vi "UMLEditor_OptionsDialog.vi"(1 "localVariables":T2 {"ObjectHotspots"."HotSpot"."y" format="%.2f"; "ObjectHotspots"."HotSpot"."x" format="%.2f"; "NodesBounds"."height" format="%.2f"; "NodesBounds"."width" format="%.2f"; "NodesBounds"."y" format="%.2f"; "NodesBounds"."x" format="%.2f"; "offset"."y" format="%.2f"; "offset"."x" format="%.2f"; "gridSize" format="%.2f"; "dragStartBounds"."height" format="%.2f"; "dragStartBounds"."width" format="%.2f"; "dragStartBounds"."y" format="%.2f"; "dragStartBounds"."x" format="%.2f"; "dragStartPoint"."y" format="%.2f"; "dragStartPoint"."x" format="%.2f"; "rubberBandStart"."y" format="%.2f"; "rubberBandStart"."x" format="%.2f"; "lastMousePoint"."y" format="%.2f"; "lastMousePoint"."x" format="%.2f"; "zoom" format="%.2f"}, 5 "error in (no error)":errorcluster) -> (19 "error out":errorcluster)   [LabVIEW 2020]
doc: "Helpinstructions."
uses:
  <resource>/Framework/Providers/Open_GDS/UML/UMLEditor/UMLEditor LocalVariablesType.ctl
  <resource>/Framework/Providers/Open_GDS/UML/AbstractNode_class/AbstractNode.lvclass
  <resource>/Framework/Providers/Open_GDS/UML/Graphics_class/Graphics.lvclass
  <resource>/Framework/Providers/Open_GDS/UML/Grid_class/Grid.lvclass
  <resource>/Framework/Providers/Open_GDS/UML/AbstractEdge_class/AbstractEdge.lvclass
  <resource>/Framework/Providers/Open_GDS/UML/UMLEditor/UMLEditor statesType.ctl
  <resource>/Framework/Providers/Open_GDS/UML/UMLEditor/UMLEditor tooltype.ctl
  <resource>/Framework/Providers/Open_GDS/UML/UMLEditor/UMLEditor_DiagramInfo.ctl
  <resource>/Framework/Providers/Open_GDS/UML/Graph_class/Graph.lvclass
  <resource>/Framework/Providers/Open_GDS/UML/General/Point/Point Point2D.ctl
  <resource>/Framework/Providers/Open_GDS/UML/General/Rectangle/Rectangle Rectangle2D.ctl
  <resource>/Framework/Providers/Open_GDS/UML/UMLEditor/UMLEditor ExportType.ctl
  <resource>/Framework/Providers/Open_GDS/UML/UMLEditor/UMLEditor FlattenCommandType.ctl
  <resource>/Framework/Providers/Open_GDS/UML/UMLEditor/UMLEditor ExecuteCommandType.ctl
  <resource>/Framework/Providers/Open_GDS/UML/ContextHelp/ContextHelp_EventType.ctl
  <resource>/Framework/Providers/Open_GDS/UML/UMLEditor/UMLEditor_HotSpotData.ctl
  <resource>/Framework/Providers/Open_GDS/UML/UMLEditor/UMLEditor_HotSpotType.ctl
  <resource>/Framework/Providers/Open_GDS/UML/UmlEditor_class/EventData.ctl
  <resource>/Framework/Providers/Open_GDS/UML/UMLEditor/UMLEditor_SyncOptions.ctl
  <resource>/Framework/Providers/Open_GDS/ClassProviders/Common/File/File_StoredPathesActions.ctl
  <resource>/Framework/Providers/Open_GDS/UML/UMLEditor/UMLEditor_StoredPathes.ctl
  <resource>/Framework/Providers/Open_GDS/UML/UMLEditor/UMLEditor_StoredColors.ctl
  <resource>/Framework/Providers/Open_GDS/ClassProviders/Common/CommonVIs/CommonVIs_ColorMemoryAction.ctl
  <resource>/Framework/Providers/Open_GDS/UML/ClassNode_class/ClassNode.lvclass
  C:/Program Files (x86)/National Instruments/LabVIEW 2020/resource/Framework/Providers/Open_GDS/UML/AbstractNode_class/AbstractNode.lvclass
  <resource>/Framework/Providers/Open_GDS/UML/ContextHelp/ContextHelp_HelpTexts.ctl
  <resource>/Framework/Providers/Open_GDS/UML/ClassNode_class/ExternalSetTypes.ctl
  <resource>/Framework/Providers/Open_GDS/UML/UmlEditor_class/UmlEditor.lvclass
panel:
  out "TabLabel":string
  out "Tab":enum32{"Color", "Paths", "General", "AutoSync"}(tab)
  in  "Class background color for <<Interface>> Stereotypes":u32(colorbox)
  in  "Default class background":u32(colorbox)
  in  "Class background with path property defined":u32(colorbox)
  in  "Class background color for <<Application/VI>> Stereotypes":u32(colorbox)
  in  "Class background color for <<TYPE/ENUM>> Stereotype":u32(colorbox)
  in  "State Background Color":u32(colorbox)
  in  "UseProjectPath":bool
  in  "ClassBasePath":path caption="Class Base Path\n(Used when releative class pathes is used)"
  in  "Classes":string(tree) caption="These classes could be converted to use a relative path"
  in  "Convert":bool
  in  "VIPath":path caption="Stereotype <<VI>>"
  in  "ApplicationPath":path caption="Stereotype <<Application>> template file"
  in  "NewFilterName":string
  in  "Filter":u16(ring) items=["Custom", "Actore Framework", "-", "Save current filter..."]
  in  "SyncOption":T1
  in  "OpenLastSavedDiagram":bool
  in  "Max number of undo steps":i32=4 min=4 max=20
  in  "ActivateUndo":bool
  in  "Classes to ignore in sychronization":string[][](table)
  in  "Attributes to ignore in sychronization":string[][](table)
  in  "CreateTypes":bool
  in  "_DeleteFilter":bool
  in  "AutoSync":u32=1 caption="Auto Synchronize diagram from source every (s)" min=1 max=3600
  in  "OptionTree":string(tree)
  in  "Help":bool
  out "ClassArray":string[](array[string])
  out "RefArray":refnum<class "AbstractNode.lvclass">[](array[class])
  in  "OK":bool
  in  "Cancel":bool
  # "Class nodes in class diagrams"
  # "State nodes in state diagrams"
  # "Template file"
  # "Note. Empty VIs will be used if template file paths are empty"
  # "Synchronization options for\nclasses and VIs"
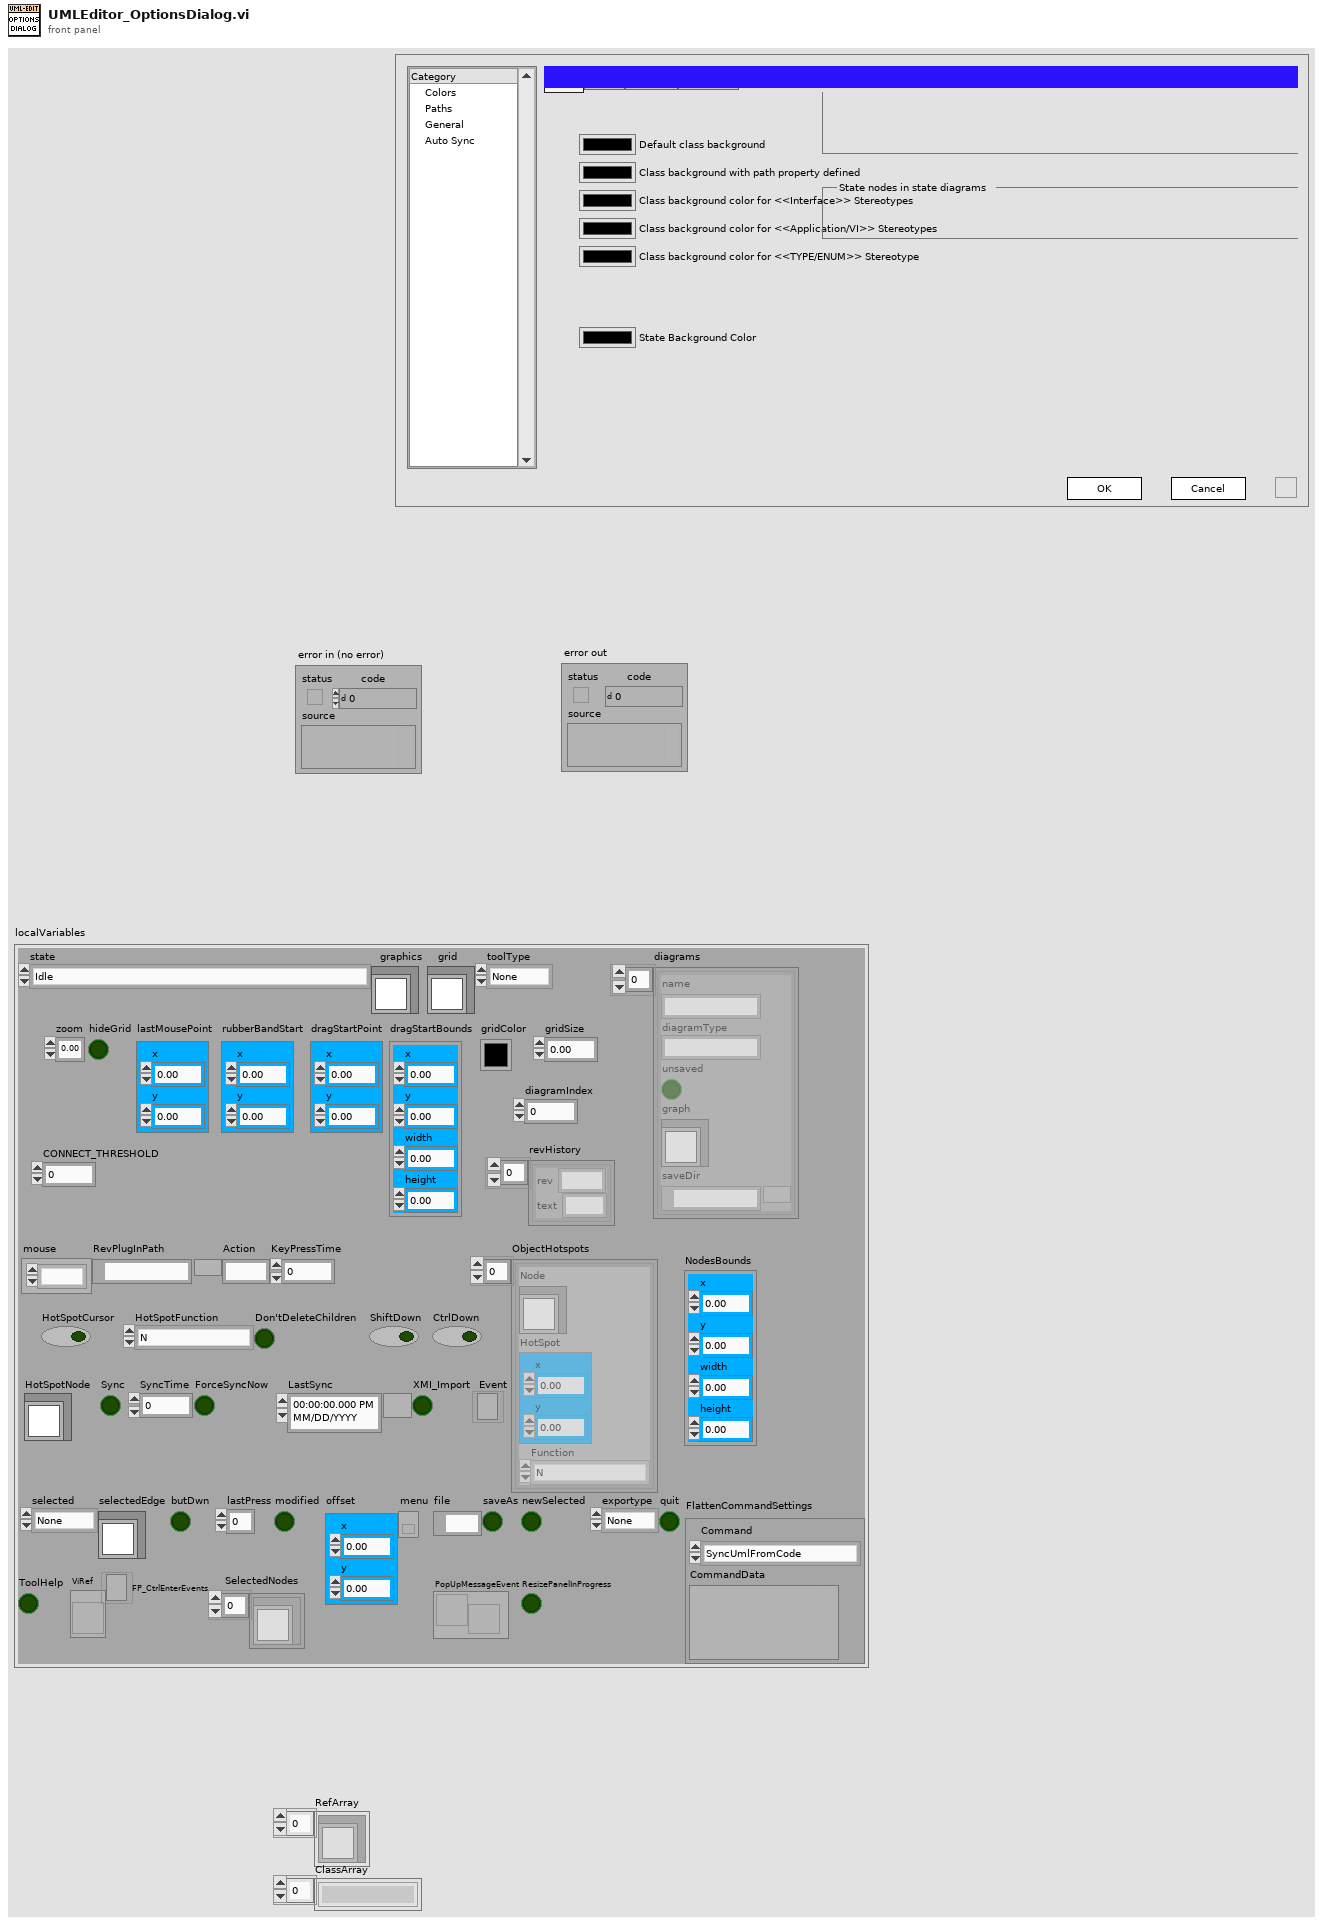
[diagram p1: front panel]
types:
  T1 = typedef "UMLEditor_SyncOptions.ctl" = cluster{"IgnoreInstrLib":bool, "IgnoreUserLib":bool, "IgnoreViLib":bool}
  T2 = typedef "UMLEditor LocalVariablesType.ctl" = cluster{"state":T3, "graphics":refnum<class "Graphics.lvclass">, "grid":refnum<class "Grid.lvclass">, "toolType":T4, "diagramIndex":i32, "diagrams":T5[], "zoom":dbl, "hideGrid":bool, "lastMousePoint":T6, "rubberBandStart":T6, "dragStartPoint":T6, "dragStartBounds":T7, "gridColor":u32, "gridSize":dbl, "CONNECT_THRESHOLD":i32, "selected":T4, "selectedEdge":refnum<class "AbstractEdge.lvclass">, "butDwn":bool, "lastPress":u32, "modified":bool, "offset":T6, "menu":refnum<k9>, "file":path, "saveAs":bool, "newSelected":bool, "exportype":T8, "quit":bool, "revHistory":cluster{"rev":string, "text":string}[], "FlattenCommandSettings":T9, "PopUpMessageEvent":T11, "ResizePanelInProgress":bool, "NodesBounds":T7, "ToolHelp":bool, "ViRef":refnum<vi>, "FP_CtrlEnterEvents":refnum<event-registration>, "SelectedNodes":refnum<class "AbstractNode.lvclass">[], "mouse":refnum<k1>, "RevPlugInPath":path, "Action":string, "KeyPressTime":u32, "ObjectHotspots":T12[], "HotSpotCursor":bool, "HotSpotFunction":T13, "Don'tDeleteChildren":bool, "ShiftDown":bool, "CtrlDown":bool, "HotSpotNode":refnum<class "AbstractNode.lvclass">, "Sync":bool, "SyncTime":u32, "ForceSyncNow":bool, "LastSync":timestamp, "XMI_Import":bool, "Event":refnum<event-registration>}
  T3 = typedef "UMLEditor statesType.ctl" = enum16{"Idle", "CheckLicense", "revHistory", "Init", "Init2", "EditSelected", "RemoveSelected", "PaintComponent", "ChangeZoom", "ChangeGridSize", "Open", "Close", "Save", "ExportPicture", "Export", "Repaint", "Error", "Exit", "QUIT", "CreateScript", "ExecuteScript", "ClassReversedEngineering", "PlugInReverseEngineering", "StateReversedEngineering", "AutoPlace", "ExecuteCommand", "OpenClass", "SyncAll", "StraightenAssociation", "Copy", "Paste", "AddNodeFromProjectTree", "AddNodeFromProjectTree+SyncAll", "PanAndRepaint", "Init3", "CopyPaste", "ApplyDesignPattern", "AnalyseViInStateDiagram", "AutoSync"}
  T4 = typedef "UMLEditor tooltype.ctl" = enum16{"None", "Node", "Edge"}
  T5 = typedef "UMLEditor_DiagramInfo.ctl" = cluster{"name":string, "diagramType":string, "unsaved":bool, "graph":refnum<class "Graph.lvclass">, "saveDir":path}
  T6 = typedef "Point Point2D.ctl" = cluster{"x":dbl, "y":dbl}
  T7 = typedef "Rectangle Rectangle2D.ctl" = cluster{"x":dbl, "y":dbl, "width":dbl, "height":dbl}
  T8 = typedef "UMLEditor ExportType.ctl" = enum16{"None", "Printer", "png", "jpg", "roseUML"}
  T9 = typedef "UMLEditor FlattenCommandType.ctl" = cluster{"Command":T10, "CommandData":variant}
  T10 = typedef "UMLEditor ExecuteCommandType.ctl" = enum16{"SyncUmlFromCode", "SyncCodeFromUML", "OpenClass", "OpenFile", "CreateClass", "CreateVI", "OpenClassAttribute", "LocateInProject", "GraphExecute"}
  T11 = typedef "ContextHelp_EventType.ctl" = refnum<user-event>
  T12 = typedef "UMLEditor_HotSpotData.ctl" = cluster{"Node":refnum<class "AbstractNode.lvclass">, "HotSpot":T6, "Function":T13}
  T13 = typedef "UMLEditor_HotSpotType.ctl" = enum16{"N", "NE", "E", "SE", "S", "SW", "W", "NW", "Expand", "Collaps"}
  T14 = typedef "UMLEditor_StoredColors.ctl" = enum16{"ClassBackgroudColor", "ClassBackgroudColorWithClassPath", "ClassBackgroudColorForApplicationVIStereotype", "ClassBackgroudColorForTypeStereotype", "StateBackgroudColor", "ClassBackgroudColorForInterfaceStereotype"}
  T15 = typedef "UMLEditor_StoredPathes.ctl" = enum16{"LastSearchPath", "QueuedArrayStateVI", "ClassBasePath", "ViTemplatePath", "ApplicationTemplatePath", "IniFilePath", "WizDir", "RevPlugInPath"}
  T16 = typedef "File_StoredPathesActions.ctl" = enum16{"Get Path", "Set Path", "Delete Path", "Clear All Paths"}
  T17 = cluster{"reference out":refnum<class "AbstractNode.lvclass">, "className":string, string, string}[]
  T18 = cluster{"reference out":refnum<class "ClassNode.lvclass">, "className":string, string, string}
  T19 = typedef "ContextHelp_HelpTexts.ctl" = enum16{"None(Hide)", "Default", "Help", "Welcome", "GettingStarted", "ClassDiagram_Help", "SequenceDiagram_Help", "UseCaseDiagram_Help", "BSelect", "BClass", "BInterface", "BPackage", "BNote", "BDependency", "BInheritance", "BInterfaceImplementation", "BAssociation", "BAggregation", "BCompAggregation", "BNoteConnector", "BObject", "BActionBar", "BCall", "BSystem", "BActor", "BUseCase", "BGeneralization", "BIncludes", "BExtends", "BUseCaseDiagramAssociation", "ClassRelationshipEdge editDialog_Bent Style", "ClassRelationshipEdge editDialog_RelationType", "ClassRelationshipEdge editDialog_Reverse association", "ClassRelationshipEdge editDialog_Start label", "ClassRelationshipEdge editDialog_Middle label", "ClassRelationshipEdge editDialog_End label", "UMLEditor reversedEngineering_Pathes", "ReversedEngineering StateReverseDialog_Help", "ReversedEngineering StateQueuedSettings_Help", "UMLEditor reversedEngineering_AddTopVIs", "UMLEditor reversedEngineering_AddClasses", "UMLEditor reversedEngineering_AddDirs", "UMLEditor reversedEngineering_Recursively", "UMLEditor reversedEngineering_Remove", "UMLEditor reversedEngineering_ClearList", "UMLEditor reversedEngineering_HideSubAss", "UMLEditor reversedEngineering_CreateTypes", "UMLEditor reversedEngineering_OnlyInheritance", "UMLEditor reversedEngineering_CreateApplication", "UMLEditor reversedEngineering_OK", "UMLEditor reversedEngineering_Cancel", "UMLEditor reversedEngineering_Help", "UMLEditor createWizardScriptFile_ScriptfilePath", "UMLEditor createWizardScriptFile_ClassPath", "UMLEditor createWizardScriptFile_Use", "UMLEditor createWizardScriptFile_PrivateDirName", "UMLEditor createWizardScriptFile_DirAppend", "UMLEditor createWizardScriptFile_Separator Character", "UMLEditor createWizardScriptFile_OK", "UMLEditor createWizardScriptFile_Cancel", "UMLEditor createWizardScriptFile_Help", "ClassNode editDialog_Class Name", "InterfaceNode editDialog_Class Name", "ClassNode editDialog_Attribute", "ClassNode editDialog_Methods", "InterfaceNode editDialog_Methods", "ClassNode editDialog_connection", "InterfaceNode editDialog_connection", "ClassNode editDialog_StereoType", "ClassNode editDialog_ShowAttrib", "ClassNode editDialog_ShowMethods", "ClassNode editDialog_ClassPath", "ClassNode editDialog_AddAttribute", "ClassNode editDialog_AddMethod", "InterfaceNode editDialog_AddMethod", "ClassNode AttributeGuide_AttributeName", "ClassNode AttributeGuide_Array?", "ClassNode AttributeGuide_Data Type", "ClassNode AttributeGuide_RefName", "ClassNode AttributeGuide_Preview", "ClassNode AttributeGuide_OK", "ClassNode AttributeGuide_Cancel", "ClassNode MethodGuide_Visibility", "ClassNode MethodGuide_Method Name", "ClassNode MethodGuide_Preview", "ClassNode MethodGuide_OK", "ClassNode MethodGuide_Cancel", "CallNode EditCallProperties_AllButtons", "ObjectNode EditObjectlProperties_AllButtons", "ActorNode EditActorProperties_AllButtons", "UseCaseRelationshipNode EditUseCaselProperties_AllButtons", "UseCaseNode EditUseCaselProperties_AllButtons", "SystemNode EditSystemProperties_AllButtons", "ReversedEngineering UpdateAttributes_AllButtons", "StateNode editDialog_AllButtons", "StateTransition editDialog_AllButtons", "ArrangeNodes Main_Picture", "ArrangeNodes Main_Zoom", "ArrangeNodes Main_Auto Zoom", "ArrangeNodes Main_shorten", "ArrangeNodes Main_Min Length", "ArrangeNodes Main_Max Length", "ArrangeNodes Main_increase", "ArrangeNodes Main_decrease", "ArrangeNodes Main_Shake", "ArrangeNodes Main", "BState", "BInitialState", "BFinalState", "BStateTransition", "StateDiagram_Help", "StateDiagram_PropertiesAllButtons", "ReversedEngineering StateReverseDialog_ClearStates", "ReversedEngineering StateReverseDialog_UseQueuedStateMachines", "ReversedEngineering StateReverseDialog_QueuedSettings", "ReversedEngineering StateReverseDialog_SearchForVIs", "ReversedEngineering StateReverseDialog_SearchCriteria", "OptionsDialog_ClassBasePath", "OptionsDialog_VIPath", "OptionsDialog_ApplicationPath", "OptionsDialog_WizDir", "OptionsDialog_IniFilePath", "OptionsDialog_DefineColors", "OptionsDialog_Help", "OptionsDialog_CreateTypes", "ClassRelationshipEdge editDialog_SplitWire"}
  T20 = typedef "ClassNode.lvclass/ExternalSetTypes.ctl" = enum16{"Name", "Attributes", "Methods", "Position", "ShowMethods", "ShowAttributes", "ClassPath"}
  T21 = typedef "CommonVIs_ColorMemoryAction.ctl" = enum16{"Get Color", "Set Color", "Delete Color", "Clear All Colors"}
  T22 = typedef "ContextHelp_ShowType.ctl" = cluster{"Header":string, "Picture":picture, "Text":string}
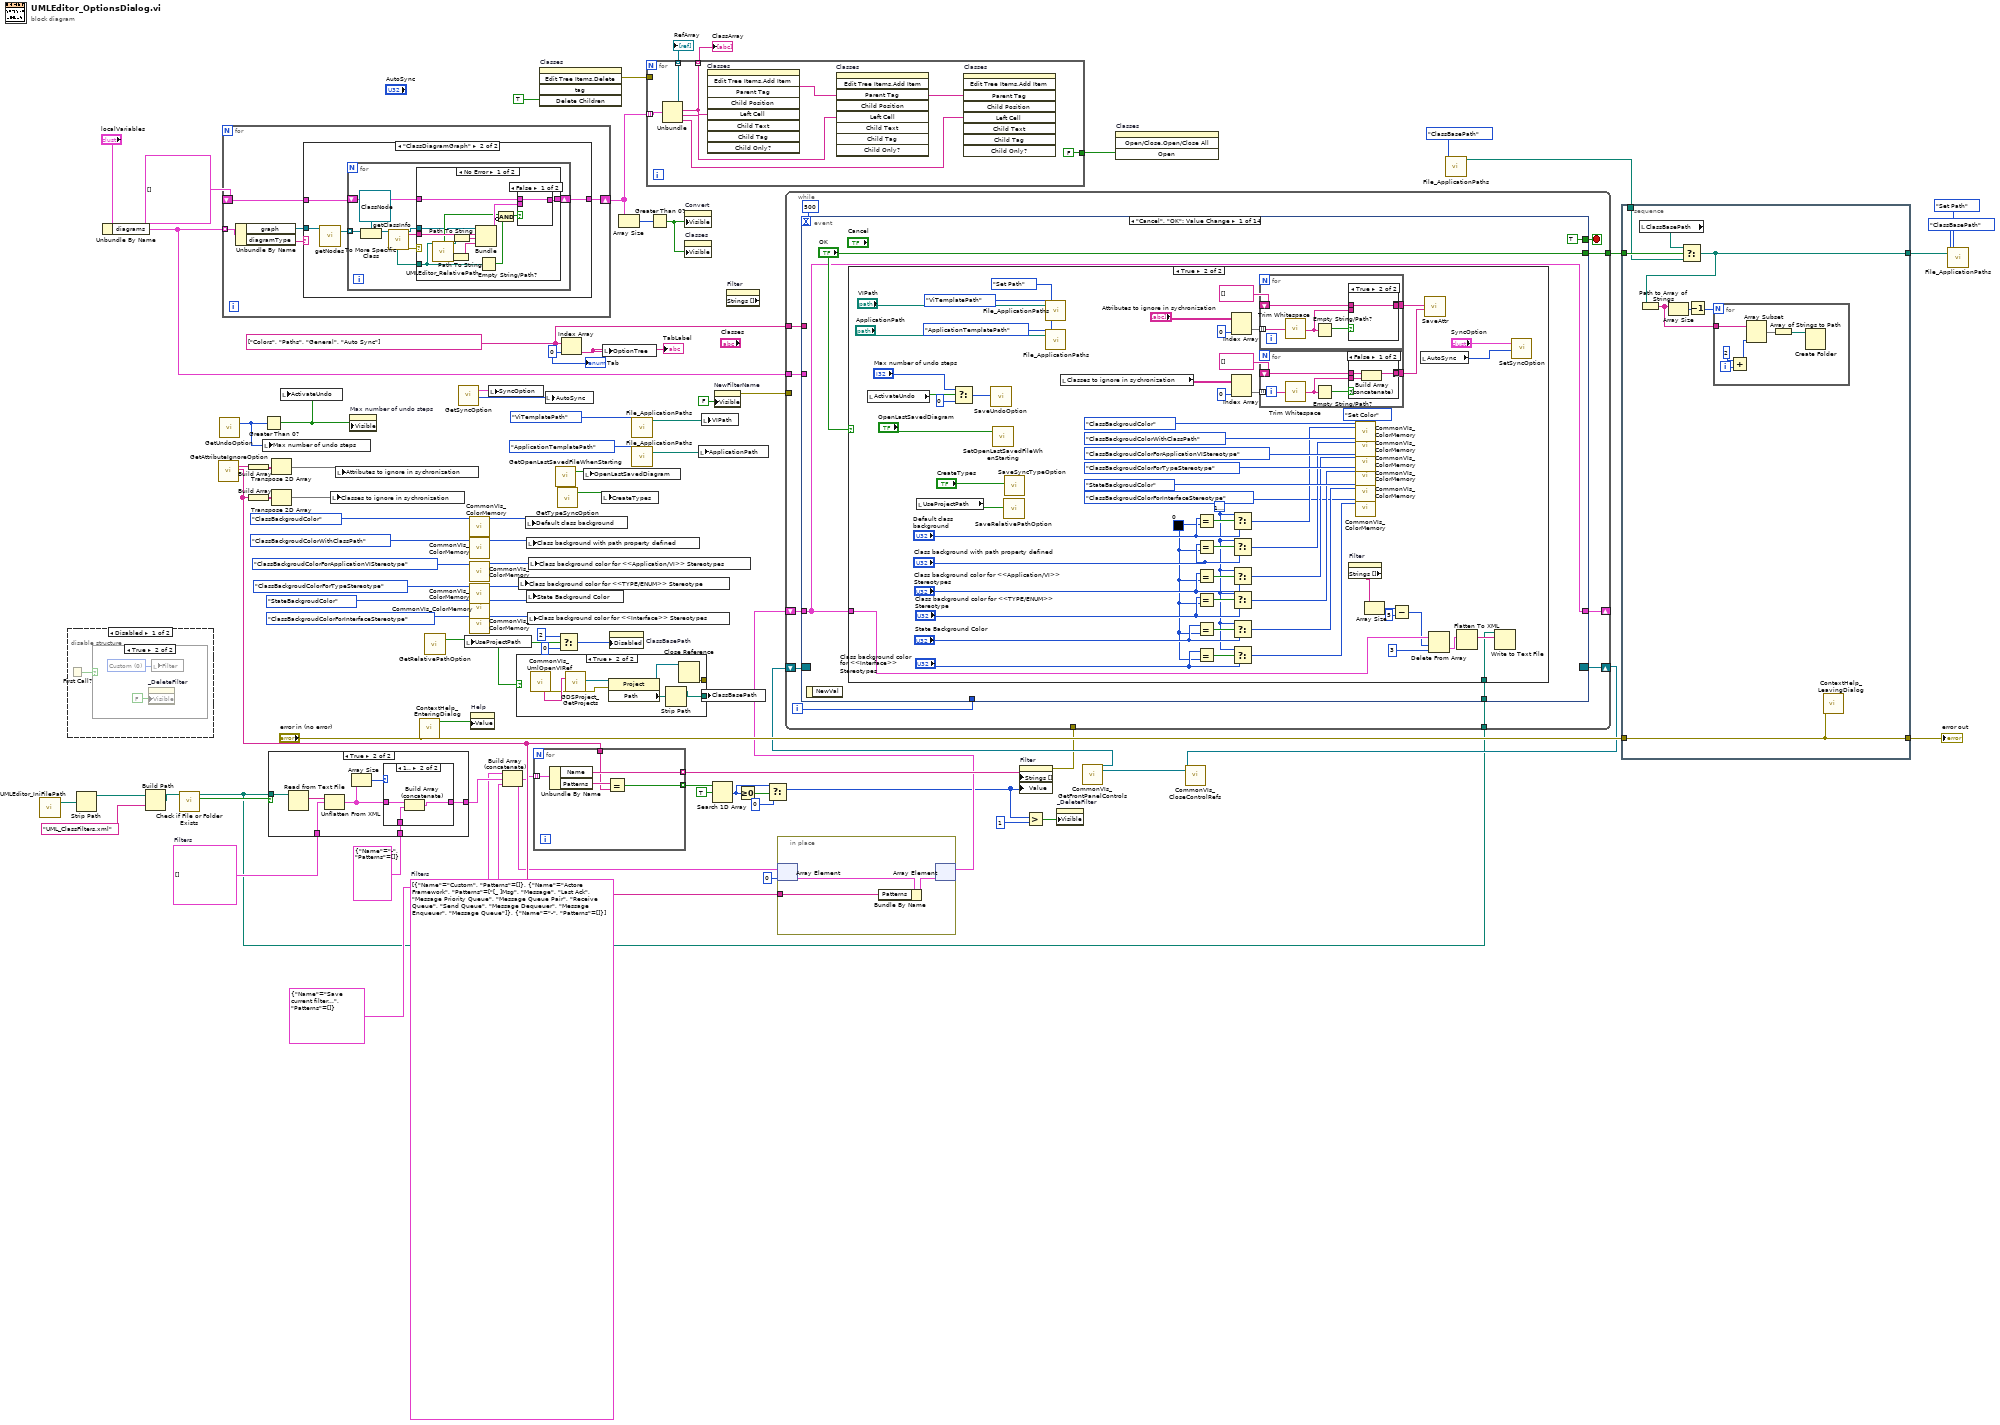
[diagram p0: block diagram]
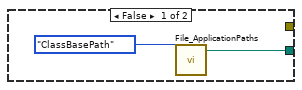
[diagram p6: hidden frame]
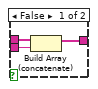
[diagram p9: hidden frame]
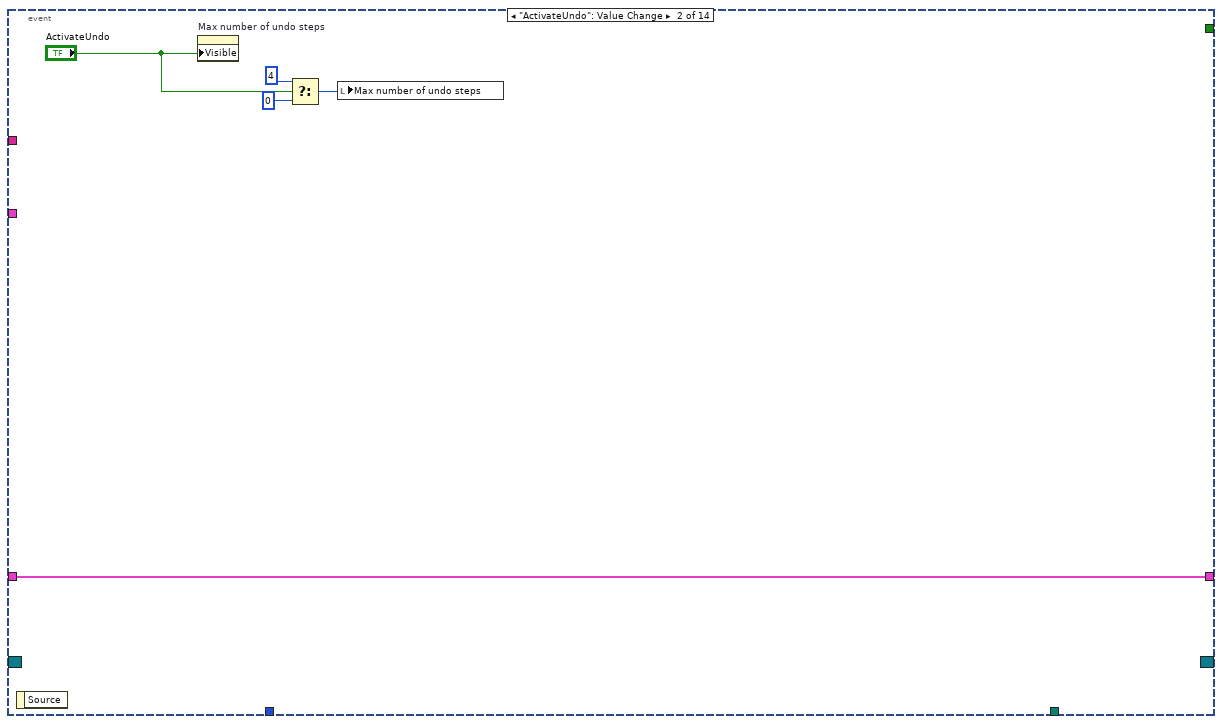
[diagram p10: hidden frame]
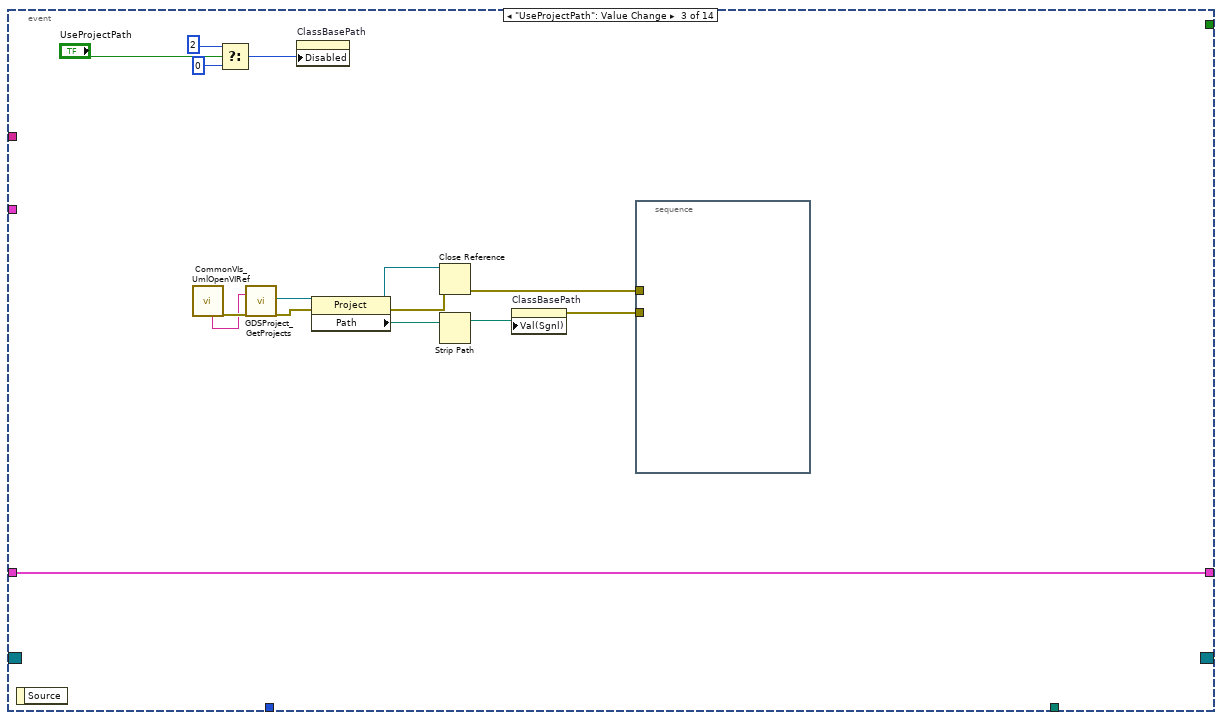
[diagram p11: hidden frame]
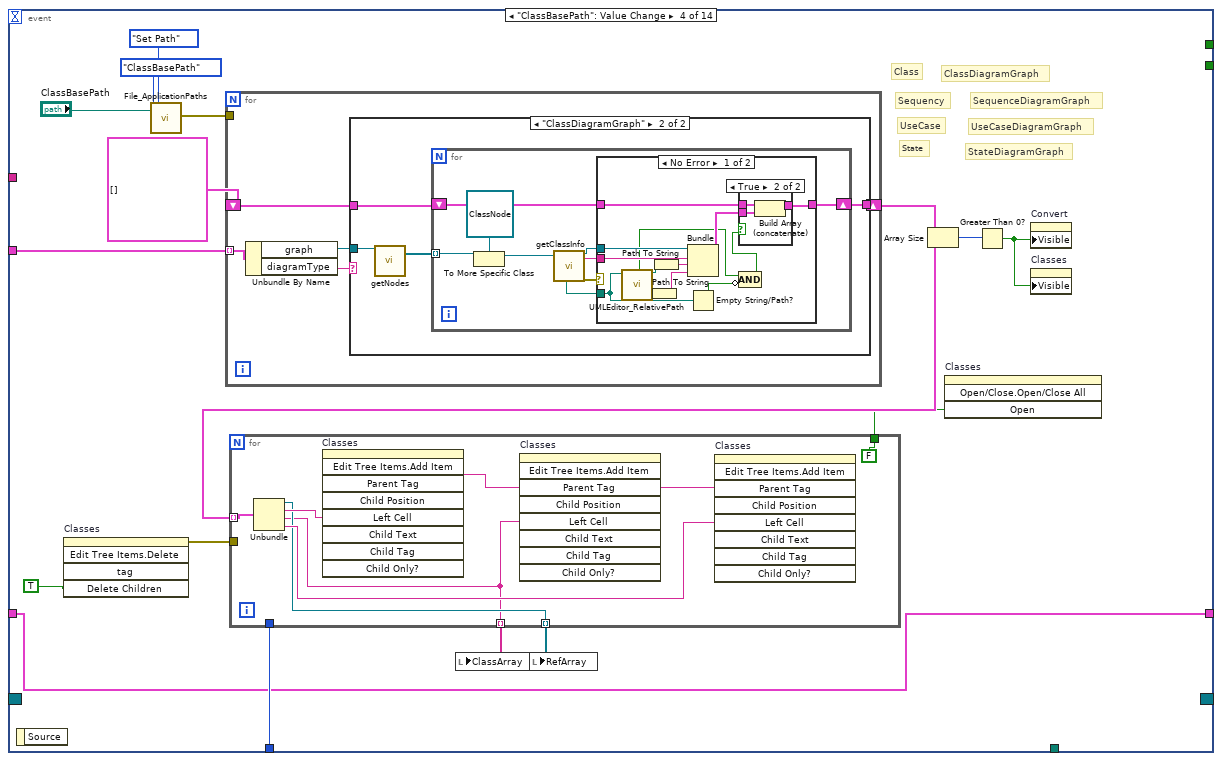
[diagram p12: hidden frame]
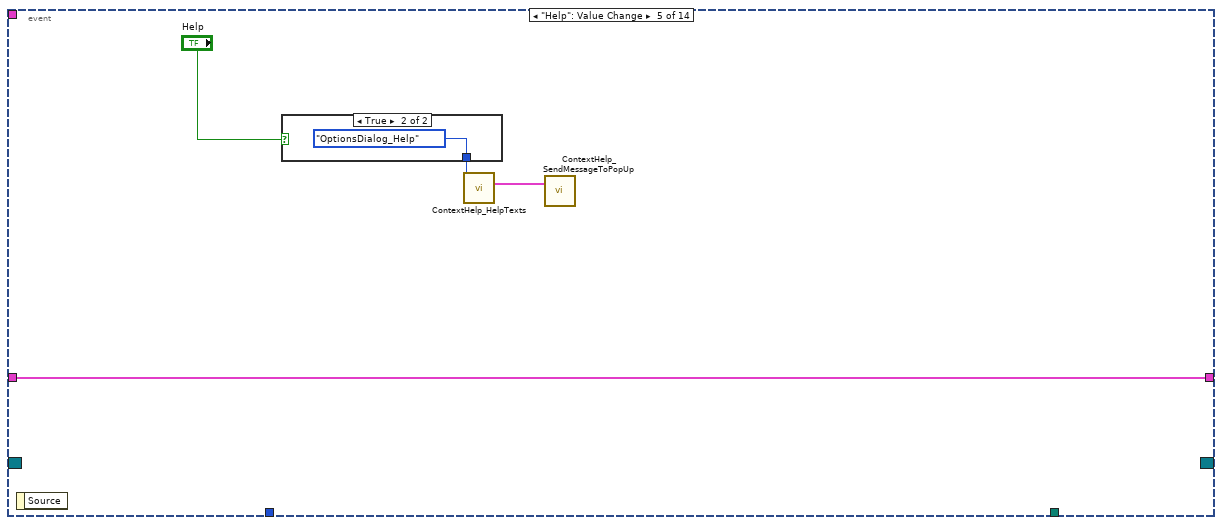
[diagram p16: hidden frame]
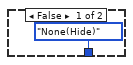
[diagram p17: hidden frame]
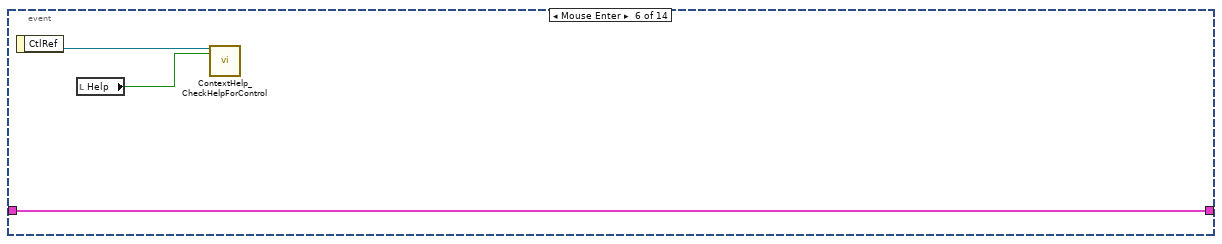
[diagram p18: hidden frame]
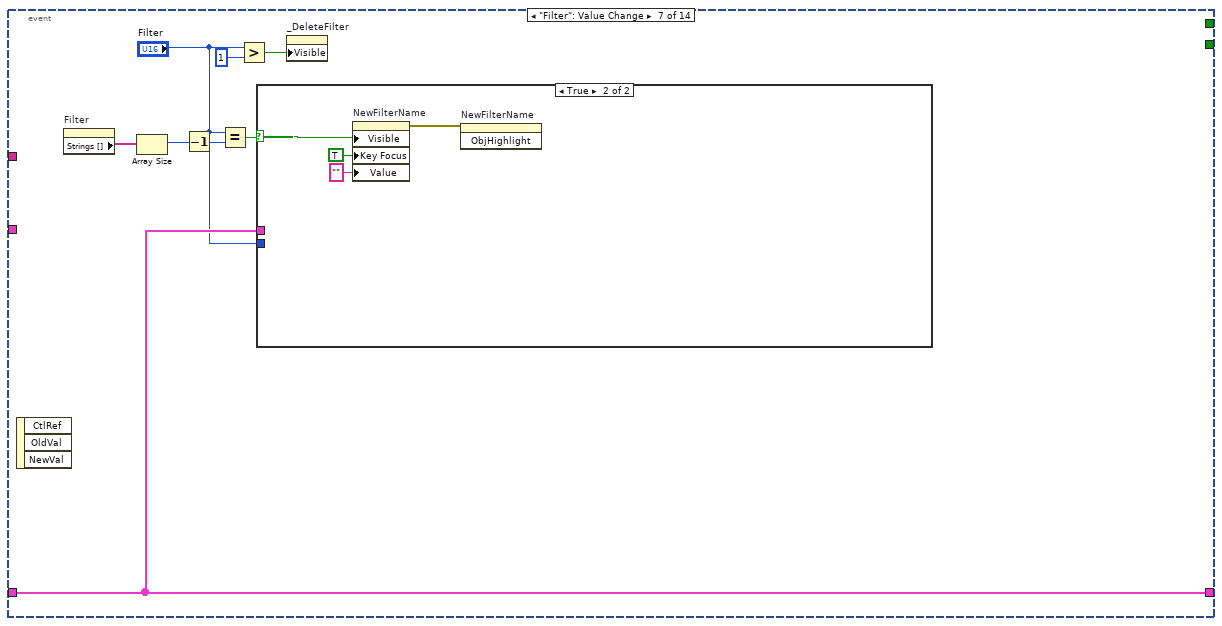
[diagram p19: hidden frame]
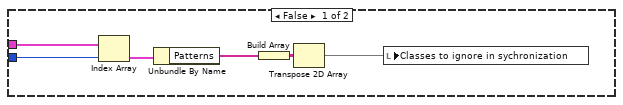
[diagram p20: hidden frame]
diagram:
  w15 = cluster{"Name":string, "Patterns":string[]}[] [{"Name"="Custom", "Patterns"=[]}, {"Name"="Actore Framework", "Patterns"=["[_ ]Msg", "Message", "Last Ack", "Message Priority Queue", "Message Queue Pair", "Receive Queue", "Send Queue", "Message Dequeuer", "Message Enqueuer", "Message Queue"]}, {"Name"="-", "Patterns"=[]}]  # Filters
  w24 = cluster{"Name":string, "Patterns":string[]}[] []  # Filters
  w56 = 0 ("index")
  w57 = string[] ["Colors", "Paths", "General", "Auto Sync"]
  n1 = call <resource>:"UMLEditor_IniFilePath.vi"() -> ("Get Path"=w29:path)  [unwired: 18 in, 1 out]
  n2 = disable-structure shown="Disabled" {
    frame Disabled {
      n3 = First Call?() -> (First Call?: T/F=w86:bool)
      n4 = case shown="True" w86 {
        frame False {
        }
        frame True {
          w88 = u16 0 items=["Custom", "Actor Framework", "-", "Save current filter as..."] ("Filter")
          n5 = property on="_DeleteFilter" class="Bool"("Visible"=FALSE) -> ()  [unwired: 2 in, 2 out]
          n6 = local write "Filter"(w88) -> ()
        }
      }
    }
    frame Enabled {
    }
  }
  n7 = Strip Path(path=w29) -> (stripped path=w28:path)  [unwired: 1 out]
  n8 = Unbundle By Name("localVariables") -> ("diagrams"=w80:T5[])
  n9 = Build Path(base path=w28, name or relative path="UML_ClassFilters.xml") -> (appended path=w26:path)
  n10 = call <vilib>:"Check if File or Folder Exists.vi"("path"=w26) -> ("file or folder exists?"=w25:bool, "dup path"=w3:path)  [unwired: 8 in, 1 out]
  n11 = call <resource>:"GetAttributeIgnoreOption.vi"() -> ("Attr"=w39:string[], "ClassesToIgnore"=w14:string[])  [unwired: 1 in, 17 out]
  n12 = call <resource>:"GetUndoOption.vi"() -> ("UndoSize"=w34:i32)  [unwired: 1 in, 18 out]
  n13 = for {
    tunnel: w80 -> [w93] mode=indexing
    shift-right: [w89] -> w82
    shift-left: T17 [] -> [w90]
    n14 = Unbundle By Name(w93) -> ("graph"=w91:refnum<class "Graph.lvclass">, "diagramType"=w92:string)
    n15 = case shown="\"ClassDiagramGraph\"" w92 {
      tunnel: w91 -> [_ w98]
      tunnel: w90 -> [w94 w96]
      tunnel: [w94 w95] -> w89
      frame "None", Default {
      }
      frame "ClassDiagramGraph" {
        n16 = call-dynamic "getNodes.vi"("reference"=w98) -> ("nodes"=w97:refnum<class "AbstractNode.lvclass">[])  [unwired: 16 in, 2 out]
        n17 = for {
          tunnel: w97 -> [w100] mode=indexing
          shift-right: [w105] -> w95
          shift-left: w96 -> [w106]
          n18 = To More Specific Class(target class=refnum<class "ClassNode.lvclass"> refnum ("reference"), reference=w100) -> (specific class reference=w99:refnum<class "ClassNode.lvclass">)  [unwired: 1 in, 1 out]
          n19 = call-dynamic "getClassInfo.vi"("reference"=w99) -> ("ClassPathUnmodified"=w102:path, "reference out"=w103:refnum<class "ClassNode.lvclass">, "className"=w104:string, "error out"=w107:errorcluster)  [unwired: 9 in, 6 out]
          n20 = case shown="No Error" w107 {
            tunnel: w106 -> [w120 w125]
            tunnel: [w119 w125] -> w105
            tunnel: w104 -> [w118 _]
            tunnel: w103 -> [w111 _]
            tunnel: w102 -> [w110 _]
            frame No Error {
              n21 = call <resource>:"UMLEditor_RelativePath.vi"("Path In"=w110) -> ("ConvertedToARelativePath"=w114:bool, "ConvertToRelativePath(If possible)"=w116:path, "ConvertToAbsolutePath(If possible)"=w117:path)  [unwired: 1 in, 15 out]
              n22 = Path To String(path=w116) -> (string=w113:string)
              n23 = Path To String(path=w117) -> (string=w112:string)
              n24 = Bundle("reference out"=w111, "className"=w118, w112, w113) -> (w115:T18)  [unwired: 1 out]
              n25 = Empty String/Path?(string/path=w110) -> (empty?=w108:bool)
              n26 = Compound Arithmetic op=AND(w114, invert w108) -> (w109:bool)
              n27 = case shown="False" w109 {
                tunnel: w120 -> [w121 w124]
                tunnel: [w121 w123] -> w119
                tunnel: w115 -> [_ w122]
                frame False {
                }
                frame True {
                  n28 = Build Array (concatenate)(w124, w122) -> (w123:T17)
                }
              }
            }
            frame Error {
            }
          }
        }
      }
    }
  }
  n29 = Build Array(w39) -> (w38:string[][])
  n30 = Build Array(w14) -> (w36:string[][])
  n31 = local write "Max number of undo steps"(w34) -> ()
  n32 = Greater Than 0?(x=w34) -> (x > 0?=w33:bool)
  n33 = case shown="True" w25 {
    tunnel: w3 -> [_ w132]
    tunnel: w24 -> [_ w130]
    tunnel: [_ w127] -> w23
    tunnel: cluster{"Name":string, "Patterns":string[]} {"Name"="-", "Patterns"=[]} ("Filter") -> [_ w126]
    frame False {
    }
    frame True {
      n34 = Read from Text File(file (use dialog)=w132) -> (text=w131:string)  [unwired: 3 in, 3 out]
      n35 = Unflatten From XML(xml string=w131, type=w130) -> (value=w128:cluster{"Name":string, "Patterns":string[]}[])  [unwired: 1 in, 1 out]
      n36 = Array Size(array=w128) -> (size(s)=w129:i32)
      n37 = case shown="1.." w129 {
        tunnel: w128 -> [w133 w136]
        tunnel: [w133 w135] -> w127
        tunnel: w126 -> [_ w134]
        frame 0, Default {
        }
        frame 1.. {
          n38 = Build Array (concatenate)(w136, w134) -> (w135:cluster{"Name":string, "Patterns":string[]}[])
        }
      }
    }
  }
  n39 = Transpose 2D Array(2D array=w38) -> (transposed array=w37:string[][])
  n40 = Transpose 2D Array(2D array=w36) -> (transposed array=w35:string[][])
  n41 = local write "ActivateUndo"(w33) -> ()
  n42 = local write "Classes to ignore in sychronization"(w35) -> ()
  n43 = local write "Attributes to ignore in sychronization"(w37) -> ()
  n44 = property on="Max number of undo steps" class="DigNum (strict)"("Visible"=w33) -> ()  [unwired: 2 in, 2 out]
  n45 = call <resource>:"ContextHelp_EnteringDialog.vi"("error in (no error)"="error in (no error)") -> ("HelpStatus"=w64:bool)  [unwired: 2 in, 16 out]
  n46 = call <resource>:"GetRelativePathOption.vi"() -> ("UseProjectFolderAsBasePath"=w41:bool)  [unwired: 1 in, 18 out]
  n47 = call <resource>:"GetSyncOption.vi"() -> ("SyncOption"=w31:T1, "SyncTime(s)"=w30:i32)  [unwired: 17 in, 1 out]
  n48 = local write "UseProjectPath"(w41) -> ()
  n49 = call <resource>:"CommonVIs_ColorMemory.vi"("ColorName"=UMLEditor_StoredColors."ClassBackgroudColor" ("UMLPathes")) -> ("Color Out"=w50:u32)  [unwired: 3 in, 15 out]
  n50 = call <resource>:"CommonVIs_ColorMemory.vi"("ColorName"=UMLEditor_StoredColors."ClassBackgroudColorWithClassPath" ("UMLPathes")) -> ("Color Out"=w49:u32)  [unwired: 3 in, 15 out]
  n51 = call <resource>:"CommonVIs_ColorMemory.vi"("ColorName"=UMLEditor_StoredColors."ClassBackgroudColorForApplicationVIStereotype" ("UMLPathes")) -> ("Color Out"=w48:u32)  [unwired: 3 in, 15 out]
  n52 = call <resource>:"CommonVIs_ColorMemory.vi"("ColorName"=UMLEditor_StoredColors."ClassBackgroudColorForTypeStereotype" ("UMLPathes")) -> ("Color Out"=w47:u32)  [unwired: 3 in, 15 out]
  n53 = call <resource>:"CommonVIs_ColorMemory.vi"("ColorName"=UMLEditor_StoredColors."StateBackgroudColor" ("UMLPathes")) -> ("Color Out"=w46:u32)  [unwired: 3 in, 15 out]
  n54 = call <resource>:"CommonVIs_ColorMemory.vi"("ColorName"=UMLEditor_StoredColors."ClassBackgroudColorForInterfaceStereotype" ("UMLPathes")) -> ("Color Out"=w2:u32)  [unwired: 3 in, 15 out]
  n55 = property on="Help" class="Bool (strict)"("Value"=w64) -> ()  [unwired: 2 in, 2 out]
  n56 = local write "SyncOption"(w31) -> ()
  n57 = Build Array (concatenate)(w15, w23, cluster{"Name":string, "Patterns":string[]} {"Name"="Save current filter...", "Patterns"=[]} ("Filter")) -> (w4:cluster{"Name":string, "Patterns":string[]}[])
  n58 = case shown="True" w41 {
    tunnel: [w137 w141] -> w42
    tunnel: [_ w139] -> _
    frame False {
      n59 = call <resource>:"File_ApplicationPaths.vi"("PathName"=UMLEditor_StoredPathes."ClassBasePath" ("UMLPathes")) -> ("Path Out"=w137:path)  [unwired: 3 in, 15 out]
    }
    frame True {
      n60 = call <resource>:"CommonVIs_UmlOpenVIRef.vi"() -> ("error out"=w145:errorcluster, "ProjectNameOut"=w146:string)  [unwired: 4 in, 6 out]
      n61 = call <resource>:"GDSProject_GetProjects.vi"("GetProjectRefByName"=w146, "error in (no error)"=w145) -> ("Project Refnum"=w143:refnum<vi>, "error out"=w144:errorcluster)  [unwired: 1 in, 15 out]
      n62 = property class="Project"(reference=w143, error in=w144) -> (reference out=w140:refnum<vi>, "Path"=w142:path)  [unwired: 1 out]
      n63 = Strip Path(path=w142) -> (stripped path=w141:path)  [unwired: 1 out]
      n64 = Close Reference(reference=w140) -> (error out=w139:errorcluster)  [unwired: 1 in]
    }
  }
  n65 = local write "Class background color for <<TYPE/ENUM>> Stereotype"(w47) -> ()
  n66 = local write "Default class background"(w50) -> ()
  n67 = local write "Class background with path property defined"(w49) -> ()
  n68 = local write "State Background Color"(w46) -> ()
  n69 = local write "Class background color for <<Interface>> Stereotypes"(w2) -> ()
  n70 = local write "Class background color for <<Application/VI>> Stereotypes"(w48) -> ()
  n71 = for {
    tunnel: w4 -> [w151] mode=indexing
    tunnel: [w150] -> w22 mode=indexing
    tunnel: w14 -> [w148]
    tunnel: [w147] -> w20 mode=indexing
    n72 = Unbundle By Name(w151) -> ("Name"=w150:string, "Patterns"=w149:string[])
    n73 = Equal?(x=w149, y=w148) -> (x = y?=w147:bool)
  }
  n74 = invoke on="Classes" class="Tree (strict)" method="Edit Tree Items.Delete"("Delete Children"=TRUE) -> (error out=w72:errorcluster)  [unwired: 4 in, 4 out]
  n75 = local write "AutoSync"(w30) -> ()
  n76 = call <resource>:"GetOpenLastSavedFileWhenStarting.vi"() -> ("OpenLastSavedFileWhenStarting"=w32:bool)  [unwired: 18 in, 1 out]
  n77 = call <resource>:"GetTypeSyncOption.vi"() -> ("TypeSyncOption"=w40:bool)  [unwired: 1 in, 18 out]
  n78 = Select(t=u8 2 ("Disabled"), s=w41, f=u8 0) -> (s? t:f=w45:u8)
  n79 = Index Array(array=w57, index=w56) -> (element=w58:string)
  "TabLabel" <- w58
  n80 = local write "OpenLastSavedDiagram"(w32) -> ()
  n81 = local write "CreateTypes"(w40) -> ()
  n82 = local write "OptionTree"(w58) -> ()
  n83 = property on="ClassBasePath" class="Path"("Disabled"=w45) -> ()  [unwired: 2 in, 2 out]
  n84 = Array Size(array=w82) -> (size(s)=w84:i32)
  n85 = call <resource>:"File_ApplicationPaths.vi"("PathName"=UMLEditor_StoredPathes."ViTemplatePath" ("UMLPathes")) -> ("Path Out"=w65:path)  [unwired: 3 in, 15 out]
  n86 = call <resource>:"File_ApplicationPaths.vi"("PathName"=UMLEditor_StoredPathes."ApplicationTemplatePath" ("UMLPathes")) -> ("Path Out"=w66:path)  [unwired: 3 in, 15 out]
  n87 = for {
    tunnel: w82 -> [w158] mode=indexing
    tunnel: w72 -> [_]
    tunnel: [FALSE ("Open")] -> w71
    tunnel: [w153] -> w70 mode=indexing
    tunnel: [w152] -> w69 mode=indexing
    n88 = Unbundle(w158) -> ("reference out"=w153:refnum<class "AbstractNode.lvclass">, "className"=w152:string, w155:string, w156:string)
    n89 = invoke on="Classes" class="Tree (strict)" method="Edit Tree Items.Add Item"("Left Cell"=w152) -> ("Edit Tree Items:Add Item"=w157:string)  [unwired: 8 in, 8 out]
    n90 = invoke on="Classes" class="Tree (strict)" method="Edit Tree Items.Add Item"("Parent Tag"=w157, "Left Cell"=w155) -> ()  [unwired: 7 in, 9 out]
    n91 = invoke on="Classes" class="Tree (strict)" method="Edit Tree Items.Add Item"("Parent Tag"=w157, "Left Cell"=w156) -> ()  [unwired: 7 in, 9 out]
  }
  "RefArray" <- w70
  "ClassArray" <- w69
  n92 = Greater Than 0?(x=w84) -> (x > 0?=w83:bool)
  n93 = property on="Convert" class="Bool"("Visible"=w83) -> ()  [unwired: 2 in, 2 out]
  n94 = property on="Classes" class="Tree (strict)"("Visible"=w83) -> ()  [unwired: 2 in, 2 out]
  n95 = local write "ApplicationPath"(w66) -> ()
  n96 = local write "VIPath"(w65) -> ()
  n97 = local write "ClassBasePath"(w42) -> ()
  n98 = Search 1D Array(1D array=w20, element=TRUE) -> (index of element=w17:i32)  [unwired: 1 in]
  n99 = property on="NewFilterName" class="Str"("Visible"=FALSE) -> (error out=w5:errorcluster)  [unwired: 2 in, 1 out]
  n100 = property on="Filter" class="Ring (strict)" props=["Strings []"]() -> ()  [unwired: 2 in, 3 out]
  n101 = Greater Or Equal To 0?(x=w17) -> (x >= 0?=w18:bool)
  n102 = Select(t=w17, s=w18, f=0) -> (s? t:f=w10:i32)
  n103 = in-place {
    in-place-border: w14 -> [w159]
    n104 = in-place-array #1(w4, 0) -> (w161:cluster{"Name":string, "Patterns":string[]})
    n105 = Bundle By Name(cluster=w161, "Patterns"=w159) -> (w160:cluster{"Name":string, "Patterns":string[]})
    n106 = in-place-array #1(w160) -> (w13:cluster{"Name":string, "Patterns":string[]}[])  [unwired: 1 out]
  }
  n107 = property on="Filter" class="Ring (strict)"("Strings []"=w22, "Value"=w10) -> (error out=w21:errorcluster)  [unwired: 2 in, 1 out]
  n108 = Greater?(x=w10, y=u16 1) -> (0:w12:bool)
  n109 = property on="_DeleteFilter" class="Bool"("Visible"=w12) -> ()  [unwired: 2 in, 2 out]
  n110 = call <resource>:"CommonVIs_GetFrontPanelControls.vi"() -> ("Event Registration Refnum"=w59:refnum<event-registration>, "ControlRefs"=w61:refnum<vi>[])  [unwired: 2 in, 16 out]
  n111 = while {
    tunnel: [w172] -> w77
    tunnel: w80 -> [w170]
    shift-right: [w168] -> w60
    shift-left: w59 -> [w167]
    tunnel: w57 -> [w165]
    tunnel: w21 -> [_]
    shift-right: [w163] -> _
    shift-left: w13 -> [w164]
    tunnel: w5 -> [_]
    tunnel: w3 -> [w162]
    i -> [w169]
    stop <- w171 stop-if-true
    n112 = event shown="[0] \"Cancel\", \"OK\": Value Change" {
      selector: w167 -> [_ _ _ _ _ _ _ _ _ _ _ _ _ _]
      dyn-events: [_ _ _ _ _ _ _ _ _ _ _ _ _ _] -> w168
      timeout: 500 -> [_ _ _ _ _ _ _ _ _ _ _ _ _ _]
      tunnel: ["OK" _ _ _ _ _ _ _ _ _ _ TRUE _ _] -> w172
      tunnel: [TRUE _ _ _ _ _ _ _ _ _ _ _ _ w454] -> w171
      tunnel: w170 -> [_ _ _ w288 _ _ _ _ _ _ _ _ _ _]
      tunnel: w169 -> [_ _ _ w276 _ _ _ _ _ _ _ _ _ _]
      tunnel: w165 -> [_ _ _ _ _ _ _ _ _ _ w437 _ _ _]
      tunnel: w164 -> [w174 w255 w260 w275 w335 w341 w345 w363 w396 w415 w434 w441 w452 w455]
      tunnel: [w174 w255 w260 w275 w335 w341 w345 w362 w396 w414 w434 w441 w452 w455] -> w163
      tunnel: w162 -> [w173 _ _ _ _ _ _ _ _ _ _ _ _ _]
      event "Cancel", "OK": Value Change {
        n113 = event-data() -> ()  [unwired: 2 out]
        n114 = case shown="True" "OK" {
          tunnel: w174 -> [_ w191]
          tunnel: w173 -> [_ w184]
          frame False {
          }
          frame True {
            w178 = u32 16777216
            w179 = u32 0
            w226 = CommonVIs_ColorMemoryAction."Set Color" ("Method (Get Color)")
            w232 = File_StoredPathesActions."Set Path" ("Method (Get Path)")
            n115 = local read "ActivateUndo"() -> (w199:bool)
            n116 = local read "UseProjectPath"() -> (w225:bool)
            n117 = Select(t="Max number of undo steps", s=w199, f=0) -> (s? t:f=w197:i32)
            n118 = call <resource>:"SaveUndoOption.vi"("UndoSize"=w197) -> ()  [unwired: 1 in, 18 out]
            n119 = call <resource>:"SetOpenLastSavedFileWhenStarting.vi"("OpenLastSavedFileWhenStarting"="OpenLastSavedDiagram") -> ()  [unwired: 18 in, 1 out]
            n120 = call <resource>:"SaveRelativePathOption.vi"("UseProjectFolderAsBasePath"=w225) -> ()  [unwired: 1 in, 18 out]
            n121 = call <resource>:"SaveSyncTypeOption.vi"("TypeSyncOption"="CreateTypes") -> ()  [unwired: 1 in, 18 out]
            n122 = call <resource>:"File_ApplicationPaths.vi"("PathName"=UMLEditor_StoredPathes."ViTemplatePath" ("UMLPathes"), "Path In"="VIPath", "Method (Get Path)"=w232) -> ()  [unwired: 1 in, 16 out]
            n123 = call <resource>:"File_ApplicationPaths.vi"("PathName"=UMLEditor_StoredPathes."ApplicationTemplatePath" ("UMLPathes"), "Path In"="ApplicationPath", "Method (Get Path)"=w232) -> ()  [unwired: 1 in, 16 out]
            n124 = local read "Classes to ignore in sychronization"() -> (w192:string[][])
            n125 = Equal?(x="Default class background", y=w179) -> (x = y?=w224:bool)
            n126 = Equal?(x="Class background with path property defined", y=w179) -> (x = y?=w221:bool)
            n127 = Equal?(x="Class background color for <<Application/VI>> Stereotypes", y=w179) -> (x = y?=w220:bool)
            n128 = Equal?(x="Class background color for <<TYPE/ENUM>> Stereotype", y=w179) -> (x = y?=w215:bool)
            n129 = Equal?(x="State Background Color", y=w179) -> (x = y?=w219:bool)
            n130 = Equal?(x="Class background color for <<Interface>> Stereotypes", y=w179) -> (x = y?=w181:bool)
            n131 = Index Array(array="Attributes to ignore in sychronization", index (col)=0 ("disabled index (col)")) -> (element=w206:string[])  [unwired: 1 in]
            n132 = Index Array(array=w192, index (col)=0 ("disabled index (col)")) -> (element=w202:string[])  [unwired: 1 in]
            n133 = Select(t=w178, s=w224, f="Default class background") -> (s? t:f=w222:u32)
            n134 = Select(t=w178, s=w221, f="Class background with path property defined") -> (s? t:f=w213:u32)
            n135 = Select(t=w178, s=w220, f="Class background color for <<Application/VI>> Stereotypes") -> (s? t:f=w212:u32)
            n136 = Select(t=w178, s=w215, f="Class background color for <<TYPE/ENUM>> Stereotype") -> (s? t:f=w211:u32)
            n137 = Select(t=w178, s=w219, f="State Background Color") -> (s? t:f=w210:u32)
            n138 = Select(t=w178, s=w181, f="Class background color for <<Interface>> Stereotypes") -> (s? t:f=w177:u32)
            n139 = for {
              tunnel: w206 -> [w250] mode=indexing
              shift-right: [w246] -> w205
              shift-left: string[] [] -> [w248]
              n140 = call <vilib>:"Trim Whitespace.vi"("string"=w250) -> ("trimmed string"=w247:string)  [unwired: 1 in]
              n141 = Empty String/Path?(string/path=w247) -> (empty?=w249:bool)
              n142 = case shown="True" w249 {
                tunnel: w248 -> [w252 w254]
                tunnel: w247 -> [w251 _]
                tunnel: [w253 w254] -> w246
                frame False {
                  n143 = Build Array (concatenate)(w252, w251) -> (w253:string[])
                }
                frame True {
                }
              }
            }
            n144 = for {
              tunnel: w202 -> [w241] mode=indexing
              shift-right: [w237] -> w200
              shift-left: string[] [] -> [w239]
              n145 = call <vilib>:"Trim Whitespace.vi"("string"=w241) -> ("trimmed string"=w238:string)  [unwired: 1 in]
              n146 = Empty String/Path?(string/path=w238) -> (empty?=w240:bool)
              n147 = case shown="False" w240 {
                tunnel: w239 -> [w243 w245]
                tunnel: w238 -> [w242 _]
                tunnel: [w244 w245] -> w237
                frame False {
                  n148 = Build Array (concatenate)(w243, w242) -> (w244:string[])
                }
                frame True {
                }
              }
            }
            n149 = property on="Filter" class="Ring (strict)"() -> ("Strings []"=w189:string[])  [unwired: 2 in, 2 out]
            n150 = call <resource>:"CommonVIs_ColorMemory.vi"("ColorName"=UMLEditor_StoredColors."ClassBackgroudColor" ("UMLPathes"), "Color In"=w222, "Method (Get Color)"=w226) -> ()  [unwired: 1 in, 16 out]
            n151 = call <resource>:"CommonVIs_ColorMemory.vi"("ColorName"=UMLEditor_StoredColors."ClassBackgroudColorWithClassPath" ("UMLPathes"), "Color In"=w213, "Method (Get Color)"=w226) -> ()  [unwired: 1 in, 16 out]
            n152 = call <resource>:"CommonVIs_ColorMemory.vi"("ColorName"=UMLEditor_StoredColors."ClassBackgroudColorForApplicationVIStereotype" ("UMLPathes"), "Color In"=w212, "Method (Get Color)"=w226) -> ()  [unwired: 1 in, 16 out]
            n153 = call <resource>:"CommonVIs_ColorMemory.vi"("ColorName"=UMLEditor_StoredColors."ClassBackgroudColorForTypeStereotype" ("UMLPathes"), "Color In"=w211, "Method (Get Color)"=w226) -> ()  [unwired: 1 in, 16 out]
            n154 = call <resource>:"CommonVIs_ColorMemory.vi"("ColorName"=UMLEditor_StoredColors."StateBackgroudColor" ("UMLPathes"), "Color In"=w210, "Method (Get Color)"=w226) -> ()  [unwired: 1 in, 16 out]
            n155 = call <resource>:"CommonVIs_ColorMemory.vi"("ColorName"=UMLEditor_StoredColors."ClassBackgroudColorForInterfaceStereotype" ("UMLPathes"), "Color In"=w177) -> ()  [unwired: 2 in, 16 out]
            n156 = Array Size(array=w189) -> (size(s)=w188:i32)
            n157 = Subtract(x=w188, y=5) -> (x-y=w186:i32)
            n158 = local read "AutoSync"() -> (w193:u32)
            n159 = call <resource>:"SaveAttr.vi"("AttrToIgnore"=w205, "ClassesToIgnore"=w200) -> ()  [unwired: 1 in, 17 out]
            n160 = Delete From Array(array=w191, length=w186, index=3) -> (deleted portion=w183:cluster{"Name":string, "Patterns":string[]}[])  [unwired: 1 out]
            n161 = Flatten To XML(6:w183) -> (2:w185:string)
            n162 = Write to Text File(file (use dialog)=w184, text=w185) -> ()  [unwired: 2 in, 3 out]
            n163 = call <resource>:"SetSyncOption.vi"("SyncOption"="SyncOption", "SyncTime(s)"=w193) -> ()  [unwired: 17 in, 1 out]
          }
        }
      }
      event "ActivateUndo": Value Change {
        n164 = event-data() -> ()  [unwired: 2 out]
        n165 = property on="Max number of undo steps" class="DigNum (strict)"("Visible"="ActivateUndo") -> ()  [unwired: 2 in, 2 out]
        n166 = Select(t=4 ("Max number of undo steps"), s="ActivateUndo", f=0) -> (s? t:f=w258:i32)
        n167 = local write "Max number of undo steps"(w258) -> ()
      }
      event "UseProjectPath": Value Change {
        n168 = event-data() -> ()  [unwired: 2 out]
        n169 = call <resource>:"CommonVIs_UmlOpenVIRef.vi"() -> ("error out"=w268:errorcluster, "ProjectNameOut"=w267:string)  [unwired: 4 in, 6 out]
        n170 = Select(t=u8 2 ("Disabled"), s="UseProjectPath", f=u8 0) -> (s? t:f=w272:u8)
        n171 = call <resource>:"GDSProject_GetProjects.vi"("GetProjectRefByName"=w267, "error in (no error)"=w268) -> ("Project Refnum"=w270:refnum<vi>, "error out"=w269:errorcluster)  [unwired: 1 in, 15 out]
        n172 = property on="ClassBasePath" class="Path"("Disabled"=w272) -> ()  [unwired: 2 in, 2 out]
        n173 = property class="Project"(reference=w270, error in=w269) -> (reference out=w264:refnum<vi>, error out=w261:errorcluster, "Path"=w266:path)
        n174 = Close Reference(reference=w264, error in (no error)=w261) -> (error out=w263:errorcluster)
        n175 = Strip Path(path=w266) -> (stripped path=w265:path)  [unwired: 1 out]
        n176 = property on="ClassBasePath" class="Path"("Val(Sgnl)"=w265) -> (error out=w262:errorcluster)  [unwired: 2 in, 1 out]
        n177 = stacked-sequence {
          tunnel: w263 -> [_]
          tunnel: w262 -> [_]
          frame #0 {
          }
        }
      }
      event "ClassBasePath": Value Change {
        # "StateDiagramGraph"
        # "SequenceDiagramGraph"
        # "UseCaseDiagramGraph"
        # "State"
        # "UseCase"
        # "Sequency"
        # "ClassDiagramGraph"
        # "Class"
        n178 = event-data() -> ()  [unwired: 2 out]
        n179 = invoke on="Classes" class="Tree (strict)" method="Edit Tree Items.Delete"("Delete Children"=TRUE) -> (error out=w280:errorcluster)  [unwired: 4 in, 4 out]
        n180 = call <resource>:"File_ApplicationPaths.vi"("PathName"=UMLEditor_StoredPathes."ClassBasePath" ("UMLPathes"), "Path In"="ClassBasePath", "Method (Get Path)"=File_StoredPathesActions."Set Path") -> ("error out"=w282:errorcluster)  [unwired: 1 in, 15 out]
        n181 = for {
          tunnel: w288 -> [w302] mode=indexing
          shift-right: [w298] -> w287
          shift-left: T17 [] -> [w299]
          tunnel: w282 -> [_]
          n182 = Unbundle By Name(w302) -> ("graph"=w300:refnum<class "Graph.lvclass">, "diagramType"=w301:string)
          n183 = case shown="\"ClassDiagramGraph\"" w301 {
            tunnel: w300 -> [_ w307]
            tunnel: w299 -> [w303 w305]
            tunnel: [w303 w304] -> w298
            frame "None", Default {
            }
            frame "ClassDiagramGraph" {
              n184 = call-dynamic "getNodes.vi"("reference"=w307) -> ("nodes"=w306:refnum<class "AbstractNode.lvclass">[])  [unwired: 16 in, 2 out]
              n185 = for {
                tunnel: w306 -> [w310] mode=indexing
                shift-right: [w314] -> w304
                shift-left: w305 -> [w315]
                n186 = To More Specific Class(target class=refnum<class "ClassNode.lvclass"> refnum ("reference"), reference=w310) -> (specific class reference=w308:refnum<class "ClassNode.lvclass">)  [unwired: 1 in, 1 out]
                n187 = call-dynamic "getClassInfo.vi"("reference"=w308) -> ("ClassPathUnmodified"=w311:path, "reference out"=w312:refnum<class "ClassNode.lvclass">, "className"=w313:string, "error out"=w316:errorcluster)  [unwired: 9 in, 6 out]
                n188 = case shown="No Error" w316 {
                  tunnel: w315 -> [w329 w334]
                  tunnel: [w328 w334] -> w314
                  tunnel: w313 -> [w327 _]
                  tunnel: w312 -> [w321 _]
                  tunnel: w311 -> [w320 _]
                  frame No Error {
                    n189 = call <resource>:"UMLEditor_RelativePath.vi"("Path In"=w320) -> ("ConvertedToARelativePath"=w318:bool, "ConvertToRelativePath(If possible)"=w325:path, "ConvertToAbsolutePath(If possible)"=w326:path)  [unwired: 1 in, 15 out]
                    n190 = Path To String(path=w325) -> (string=w323:string)
                    n191 = Path To String(path=w326) -> (string=w322:string)
                    n192 = Bundle("reference out"=w321, "className"=w327, w322, w323) -> (w324:T18)  [unwired: 1 out]
                    n193 = Empty String/Path?(string/path=w320) -> (empty?=w319:bool)
                    n194 = Compound Arithmetic op=AND(w318, invert w319) -> (w317:bool)
                    n195 = case shown="True" w317 {
                      tunnel: w329 -> [w330 w333]
                      tunnel: [w330 w332] -> w328
                      tunnel: w324 -> [_ w331]
                      frame False {
                      }
                      frame True {
                        n196 = Build Array (concatenate)(w333, w331) -> (w332:T17)
                      }
                    }
                  }
                  frame Error {
                  }
                }
              }
            }
          }
        }
        n197 = for {
          tunnel: w287 -> [w297] mode=indexing
          tunnel: [w293] -> w277 mode=indexing
          tunnel: [w292] -> w278 mode=indexing
          tunnel: w280 -> [_]
          tunnel: [FALSE ("Open")] -> w279
          tunnel: w276 -> [_]
          n198 = Unbundle(w297) -> ("reference out"=w293:refnum<class "AbstractNode.lvclass">, "className"=w294:string, w292:string, w295:string)
          n199 = invoke on="Classes" class="Tree (strict)" method="Edit Tree Items.Add Item"("Left Cell"=w294) -> ("Edit Tree Items:Add Item"=w296:string)  [unwired: 8 in, 8 out]
          n200 = invoke on="Classes" class="Tree (strict)" method="Edit Tree Items.Add Item"("Parent Tag"=w296, "Left Cell"=w292) -> ()  [unwired: 7 in, 9 out]
          n201 = invoke on="Classes" class="Tree (strict)" method="Edit Tree Items.Add Item"("Parent Tag"=w296, "Left Cell"=w295) -> ()  [unwired: 7 in, 9 out]
        }
        n202 = local write "ClassArray"(w278) -> ()
        n203 = local write "RefArray"(w277) -> ()
        n204 = Array Size(array=w287) -> (size(s)=w286:i32)
        n205 = invoke on="Classes" class="Tree (strict)" method="Open/Close.Open/Close All"("Open"=w279) -> ()  [unwired: 3 in, 4 out]
        n206 = Greater Than 0?(x=w286) -> (x > 0?=w289:bool)
        n207 = property on="Convert" class="Bool"("Visible"=w289) -> ()  [unwired: 2 in, 2 out]
        n208 = property on="Classes" class="Tree (strict)"("Visible"=w289) -> ()  [unwired: 2 in, 2 out]
      }
      event "Help": Value Change {
        n209 = event-data() -> ()  [unwired: 2 out]
        n210 = case shown="True" "Help" {
          tunnel: [ContextHelp_HelpTexts."None(Hide)" ("HelpText") ContextHelp_HelpTexts."OptionsDialog_Help" ("HelpText")] -> w337
          frame False {
          }
          frame True {
          }
        }
        n211 = call <resource>:"ContextHelp_HelpTexts.vi"("HelpText (enum or string)"=w337) -> ("HelpOut"=w338:T22)  [unwired: 18 out]
        n212 = call <resource>:"ContextHelp_SendMessageToPopUp.vi"("PopUpMessage"=w338) -> ()  [unwired: 2 in, 17 out]
      }
      event Mouse Enter {
        n213 = event-data() -> ("CtlRef"=w343:refnum<vi>)  [unwired: 1 out]
        n214 = local read "Help"() -> (w342:bool)
        n215 = call <resource>:"ContextHelp_CheckHelpForControl.vi"("Ctl Refnum"=w343, "Help"=w342) -> ()  [unwired: 1 in, 17 out]
      }
      event "Filter": Value Change {
        n216 = event-data() -> ()  [unwired: 4 out]
        n217 = property on="Filter" class="Ring (strict)"() -> ("Strings []"=w349:string[])  [unwired: 2 in, 2 out]
        n218 = Array Size(array=w349) -> (size(s)=w348:i32)
        n219 = Decrement(x=w348) -> (x-1=w347:i32)
        n220 = Equal?(x="Filter", y=w347) -> (x = y?=w346:bool)
        n221 = Greater?(x="Filter", y=u16 1) -> (0:w350:bool)
        n222 = case shown="True" w346 {
          selector: w346 -> [_ w361]
          tunnel: w345 -> [w353 _]
          tunnel: "Filter" -> [w352 _]
          frame False {
            n223 = Index Array(array=w353, index=w352) -> (element=w354:cluster{"Name":string, "Patterns":string[]})
            n224 = Unbundle By Name(w354) -> ("Patterns"=w357:string[])
            n225 = Build Array(w357) -> (w356:string[][])
            n226 = Transpose 2D Array(2D array=w356) -> (transposed array=w355:string[][])
            n227 = local write "Classes to ignore in sychronization"(w355) -> ()
          }
          frame True {
            n228 = property on="NewFilterName" class="Str"("Visible"=w361, "Key Focus"=TRUE, "Value"="" ("NewFilterName")) -> (error out=w359:errorcluster)  [unwired: 2 in, 1 out]
            n229 = invoke on="NewFilterName" class="Str" method="ObjHighlight"(error in=w359) -> ()  [unwired: 2 in, 3 out]
          }
        }
        n230 = property on="_DeleteFilter" class="Bool"("Visible"=w350) -> ()  [unwired: 2 in, 2 out]
      }
      event "NewFilterName": Value Change {
        n231 = event-data() -> ()  [unwired: 4 out]
        n232 = case shown="Default" "NewFilterName" {
          selector: "NewFilterName" -> [_ w375]
          tunnel: w363 -> [w366 w369]
          tunnel: [w366 w377] -> w362
          frame "" {
          }
          frame Default {
            n233 = property on="Filter" class="Ring (strict)"() -> ("Strings []"=w379:string[])  [unwired: 2 in, 2 out]
            n234 = local read "Classes to ignore in sychronization"() -> (w374:string[][])
            n235 = Array Size(array=w379) -> (size(s)=w380:i32)
            n236 = Subtract(x=w380, y=2) -> (x-y=w370:i32)
            n237 = case shown="2" w370 {
              selector: w370 -> [w382 w389]
              tunnel: w369 -> [w383 w387]
              tunnel: [w383 w386] -> w368
              tunnel: [w382 w388] -> w367
              frame Default {
              }
              frame 2 {
                n238 = Increment(x=w389) -> (x+1=w388:i32)
                n239 = Insert Into Array(array=w387, index=2, new element=cluster{"Name":string, "Patterns":string[]} {"Name"="-", "Patterns"=[]} ("Filter")) -> (w386:cluster{"Name":string, "Patterns":string[]}[])
              }
            }
            n240 = Index Array(array=w374, index (col)=0 ("disabled index (col)")) -> (element=w372:string[])  [unwired: 1 in]
            n241 = Bundle By Name(cluster=cluster{"Name":string, "Patterns":string[]} {"Name"="-", "Patterns"=[]} ("Filter"), "Name"=w375, "Patterns"=w372) -> (w371:cluster{"Name":string, "Patterns":string[]})
            n242 = Insert Into Array(array=w368, index=w367, new element=w371) -> (w377:cluster{"Name":string, "Patterns":string[]}[])
            n243 = for {
              tunnel: w377 -> [w390] mode=indexing
              tunnel: [w391] -> w378 mode=indexing
              n244 = Unbundle By Name(w390) -> ("Name"=w391:string)  [unwired: 1 out]
            }
            n245 = property on="Filter" class="Ring (strict)"("Strings []"=w378, "Value"=w367) -> ()  [unwired: 2 in, 2 out]
          }
        }
        n246 = property on="NewFilterName" class="Str"("Visible"=FALSE) -> ()  [unwired: 2 in, 2 out]
      }
      event "Classes to ignore in sychronization": Value Change {
        n247 = event-data() -> ()  [unwired: 4 out]
        n248 = Index Array(array="Classes to ignore in sychronization", index (col)=0 ("disabled index (col)")) -> (element=w393:string[])  [unwired: 1 in]
        n249 = for {
          tunnel: w396 -> [w406] mode=indexing
          tunnel: [w405] -> _ mode=indexing
          tunnel: w393 -> [w403]
          tunnel: [w402] -> w397 mode=indexing
          n250 = Unbundle By Name(w406) -> ("Name"=w405:string, "Patterns"=w404:string[])
          n251 = Equal?(x=w404, y=w403) -> (x = y?=w402:bool)
        }
        n252 = Search 1D Array(1D array=w397, element=TRUE) -> (index of element=w400:i32)  [unwired: 1 in]
        n253 = Greater Or Equal To 0?(x=w400) -> (x >= 0?=w399:bool)
        n254 = Select(t=w400, s=w399, f=0) -> (s? t:f=w392:i32)
        n255 = property on="Filter" class="Ring (strict)"("Value"=w392) -> ()  [unwired: 2 in, 2 out]
      }
      event "_DeleteFilter": Value Change {
        n256 = event-data() -> ()  [unwired: 4 out]
        n257 = local read "Filter"() -> (w408:u16)
        n258 = property on="Filter" class="Ring (strict)"() -> ("Strings []"=w411:string[])  [unwired: 2 in, 2 out]
        n259 = Array Size(array=w411) -> (size(s)=w410:i32)
        n260 = Decrement(x=w410) -> (x-1=w409:i32)
        n261 = Equal?(x=w408, y=w409) -> (x = y?=w407:bool)
        n262 = property on="NewFilterName" class="Str"("Visible"=FALSE) -> ()  [unwired: 2 in, 2 out]
        n263 = case shown="False" w407 {
          tunnel: w415 -> [w425 w433]
          tunnel: [w421 w433] -> w414
          tunnel: [w419 _] -> w413
          tunnel: w411 -> [w418 _]
          tunnel: w408 -> [w417 _]
          frame False {
            n264 = Delete From Array(array=w418, index=w417) -> (array with subset deleted=w423:string[])  [unwired: 1 in, 1 out]
            n265 = Delete From Array(array=w425, index=w417) -> (array with subset deleted=w422:cluster{"Name":string, "Patterns":string[]}[])  [unwired: 1 in, 1 out]
            n266 = Array Size(array=w423) -> (size(s)=w424:i32)
            n267 = case shown="5" w424 {
              tunnel: w423 -> [w427 w432]
              tunnel: [w427 w431] -> w420
              tunnel: w422 -> [w426 w430]
              tunnel: [w426 w428] -> w421
              frame 0, Default {
              }
              frame 5 {
                w429 = 2 ("index")
                n268 = Delete From Array(array=w432, index=w429) -> (array with subset deleted=w431:string[])  [unwired: 1 in, 1 out]
                n269 = Delete From Array(array=w430, index=w429) -> (array with subset deleted=w428:cluster{"Name":string, "Patterns":string[]}[])  [unwired: 1 in, 1 out]
              }
            }
            n270 = property on="Filter" class="Ring (strict)"("Strings []"=w420) -> (error out=w419:errorcluster)  [unwired: 2 in, 1 out]
          }
          frame True {
          }
        }
        n271 = property on="Filter" class="Ring (strict)"(error in=w413, "Val(Sgnl)"=u16 0 ("Value (Signaling)")) -> ()  [unwired: 1 in, 2 out]
      }
      event "OptionTree": Value Change {
        n272 = event-data() -> ()  [unwired: 7 out]
        n273 = Search 1D Array(1D array=w437, element="OptionTree") -> (index of element=w439:i32)  [unwired: 1 out]
        n274 = Max & Min(x=w439, y=0) -> (max(x,y)=w435:i32)  [unwired: 1 out]
        n275 = Index Array(array=w437, index=w435) -> (element=w436:string)
        n276 = local write "Tab"(w435) -> ()
        n277 = local write "OptionTree"(w436) -> ()
        n278 = local write "TabLabel"(w436) -> ()
      }
      event "Convert": Value Change {
        w442 = FALSE ("Visible")
        n279 = event-data() -> ()  [unwired: 2 out]
        n280 = local read "ClassArray"() -> (w445:string[])
        n281 = local read "RefArray"() -> (w444:refnum<class "AbstractNode.lvclass">[])
        n282 = for {
          tunnel: w445 -> [w449] mode=indexing
          tunnel: w444 -> [w447] mode=indexing
          n283 = String To Path(string=w449) -> (path=w450:path)
          n284 = To More Specific Class(target class=refnum<class "ClassNode.lvclass"> refnum ("reference"), reference=w447) -> (specific class reference=w446:refnum<class "ClassNode.lvclass">)  [unwired: 1 in, 1 out]
          n285 = call-dynamic "ExternalSetParam.vi"("reference"=w446, "setParameter"=ExternalSetTypes."ClassPath", "ClassPath"=w450) -> ()  [unwired: 15 in, 2 out]
        }
        n286 = property on="Convert" class="Bool"("Visible"=w442) -> ()  [unwired: 2 in, 2 out]
        n287 = property on="Classes" class="Tree (strict)"("Visible"=w442) -> ()  [unwired: 2 in, 2 out]
      }
      event Timeout {
        n288 = event-data() -> ()  [unwired: 2 out]
        n289 = property class="VI"("Front Panel Window:Is Frontmost"=TRUE) -> ()  [unwired: 2 in, 2 out]
      }
      event Panel Close? {
        w454 = TRUE ("Discard?")
        n290 = event-data() -> ()  [unwired: 2 out]
        n291 = event-data("Discard?"=w454) -> ()  [unwired: 1 in, 1 out]
      }
    }
  }
  n292 = invoke on="Classes" class="Tree (strict)" method="Open/Close.Open/Close All"("Open"=w71) -> ()  [unwired: 3 in, 4 out]
  n293 = call <resource>:"CommonVIs_CloseControlRefs.vi"("Event Registration Refnum"=w60, "ControlRefs"=w61) -> ()  [unwired: 1 in, 17 out]
  n294 = call <resource>:"File_ApplicationPaths.vi"("PathName"=UMLEditor_StoredPathes."ClassBasePath" ("UMLPathes")) -> ("Path Out"=w75:path)  [unwired: 3 in, 15 out]
  n295 = stacked-sequence {
    tunnel: w77 -> [w463]
    tunnel: w75 -> [w461]
    tunnel: [w458] -> w74
    tunnel: "error in (no error)" -> [w456]
    tunnel: [w456] -> w62
    frame #0 {
      n296 = local read "ClassBasePath"() -> (w462:path)
      n297 = Select(t=w462, s=w463, f=w461) -> (s? t:f=w458:path)
      n298 = Path to Array of Strings(0:w458) -> (2:w457:string[])  [unwired: 1 out]
      n299 = Array Size(array=w457) -> (size(s)=w460:i32)
      n300 = Decrement(x=w460) -> (x-1=w459:i32)
      n301 = for {
        N: w459 -> [_]
        tunnel: w457 -> [w466]
        i -> [w465]
        n302 = Add(x=2 ("y"), y=w465) -> (x+y=w469:i32)
        n303 = Array Subset(array=w466, length=w469) -> (w468:string[])  [unwired: 1 in]
        n304 = Array of Strings to Path(0:w468) -> (2:w464:path)  [unwired: 1 out]
        n305 = Create Folder(path (use dialog)=w464) -> ()  [unwired: 1 in, 4 out]
      }
      n306 = call <resource>:"ContextHelp_LeavingDialog.vi"("error in (no error)"=w456) -> ()  [unwired: 2 in, 17 out]
    }
  }
  "error out" <- w62
  n307 = call <resource>:"File_ApplicationPaths.vi"("PathName"=UMLEditor_StoredPathes."ClassBasePath" ("UMLPathes"), "Path In"=w74, "Method (Get Path)"=File_StoredPathesActions."Set Path") -> ()  [unwired: 1 in, 16 out]
  "Tab" <- w56
